vi "Create FIFO.vi"(8 "error in (no error)":errorcluster, 10 "number of elements":u32, 11 "Pool in":refnum<class "Pool.lvclass">) -> (0 "error out":errorcluster, 3 "Pool out":refnum<class "Pool.lvclass">)   [LabVIEW 2017, in "DSF Core.lvlib" / "Pool.lvclass"]
uses:
  Pool.lvclass
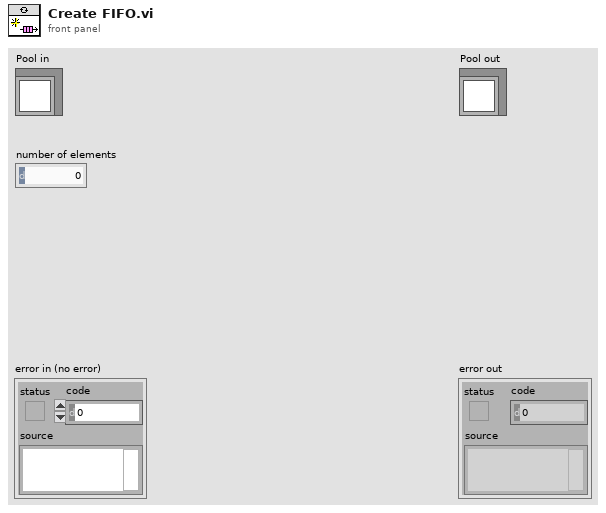
[diagram p1: front panel]
types:
  T1 = cluster{"read mode":enum16{"polling", "blocking"}, "write mode":enum16{"polling", "blocking"}}
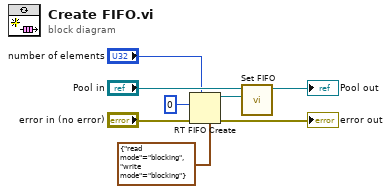
[diagram p0: block diagram]
diagram:
  n1 = RT FIFO Create(1:0, 3:"error in (no error)", 4:"number of elements", 7:T1 {"read mode"=enum."blocking", "write mode"=enum."blocking"} ("r/w modes (polling,polling)")) -> (8:w5:refnum<k33>, 11:→"error out":errorcluster)  [unwired: 4 in, 1 out]
  n2 = call "Set FIFO.vi"("FIFO"=w5, "Pool in"="Pool in") -> ("Pool out"=→"Pool out":refnum<class "Pool.lvclass">)  [unwired: 9 in]
